vi "sm u8 write array and increment.vi"(8 "error in (no error)":errorcluster, 9 "Increment value":u64=1, 10 "value in":u8[](array[numeric]), 11 "pointer in":u64) -> (0 "error out":errorcluster, 3 "Shared Memory PTR out":u64)   [LabVIEW 2018, in "linuxSharedMemory.lvlib"]
uses:
  linuxSharedMemory.lvlib
  <vilib>/NI/NI Linux RT IPC/Shared Memory/Pointer Operations/Write 1D Array U8.vi
  <vilib>/NI/NI Linux RT IPC/Shared Memory/Pointer Operations/In Place Write 1D Array U8.vi
  <vilib>/NI/NI Linux RT IPC/Shared Memory/Linux RT IPC.Shared Memory.lvlib
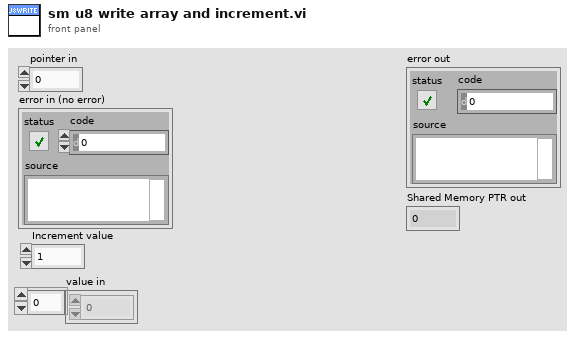
[diagram p1: front panel]
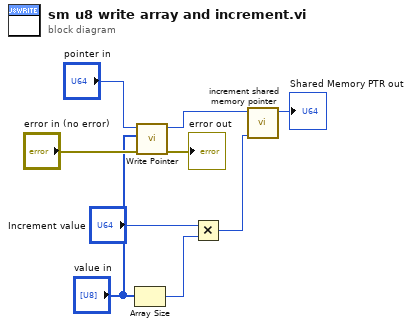
[diagram p0: block diagram]
diagram:
  n1 = Array Size(array="value in") -> (size(s)=w2:i32)
  n2 = call-poly <vilib>:"Write Pointer.vi"("error in (no error)"="error in (no error)", "value"="value in", "pointer in"="pointer in") -> ("error out"=→"error out":errorcluster, "pointer out"=w6:u64)  [unwired: 5 in, 2 out]
  n3 = Multiply(x="Increment value", y=w2) -> (x*y=w4:u64)
  n4 = call "increment shared memory pointer.vi"("Increment value"=w4, "Shared Memory PTR in"=w6) -> ("Shared Memory PTR out"=→"Shared Memory PTR out":u64)  [unwired: 9 in]
